vi "ReadTime.vi"(8 "Input":string, 9 "Status in":refnum<vi>) -> (3 "Status out":refnum<vi>)   [LabVIEW 2012, in "StimulCtrls.lvlib"]
uses:
  StimulCtrls.lvlib
panel:
  out "Current Time":string
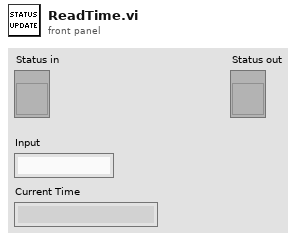
[diagram p1: front panel]
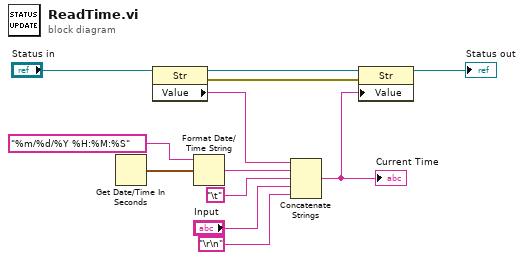
[diagram p0: block diagram]
diagram:
  n1 = Get Date/Time In Seconds() -> (seconds since 1Jan1904=w12:timestamp)
  n2 = property class="Str"(reference="Status in") -> (reference out=w3:refnum<vi>, error out=w2:errorcluster, "Value"=w5:string)  [unwired: 1 in]
  n3 = Format Date/Time String(time format string (%c)="%m/%d/%Y %H:%M:%S", seconds (now)=w12) -> (date/time string=w11:string)  [unwired: 1 in]
  n4 = Concatenate Strings(w5, w11, "\t", "Input", "\r\n") -> (w4:string)
  "Current Time" <- w4
  n5 = property class="Str"(reference=w3, error in=w2, "Value"=w4) -> (reference out=→"Status out":refnum<vi>)  [unwired: 1 out]
